vi "vipm_BuildVIPackage.vi"(8 "error in (no error)":errorcluster, 11 "CommandLine":string[](array[string])) -> (0 "error out":errorcluster, 2 "test details":string, 3 "output to action":string)   [LabVIEW 2014]
uses:
  <userlib>/_OpenG.lib/string/string.llb/Trim Whitespace (String)__ogtk.vi
  <vilib>/JKI/VIPM API/VIPM API_vipm_api.lvlib
  _lvcicd/_lvcicd_support_2014.lvlib
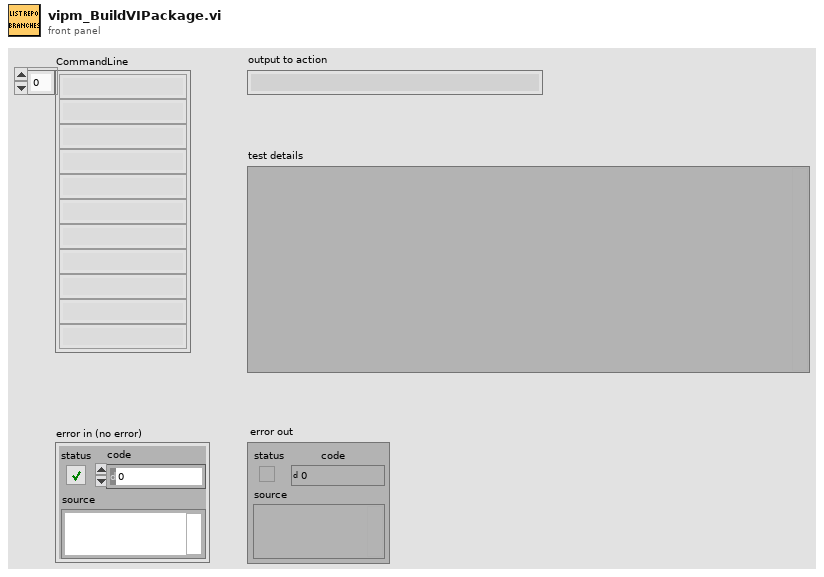
[diagram p1: front panel]
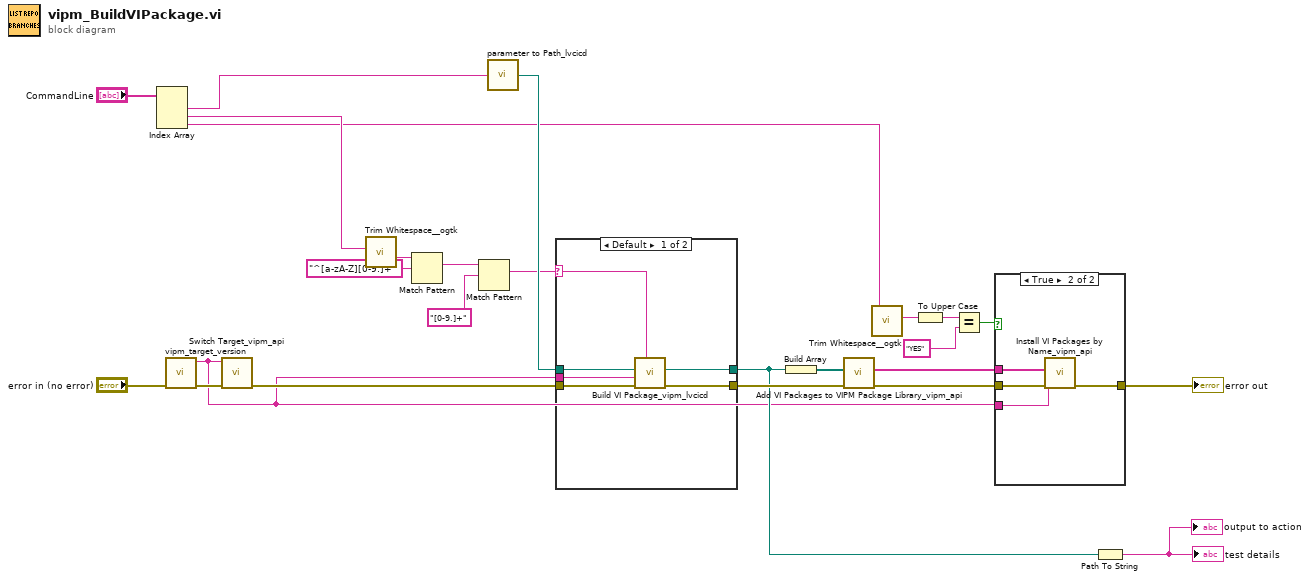
[diagram p0: block diagram]
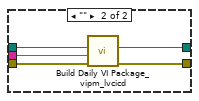
[diagram p2: hidden frame]
diagram:
  n1 = Index Array(array="CommandLine") -> (element #1=w22:string, element #2=w2:string, element #3=w1:string)  [unwired: 3 in]
  n2 = call "vipm_target_version.vi"() -> ("vipm Taget version"=w9:string)  [unwired: 11 in]
  n3 = call <vilib>:"Switch Target_vipm_api.vi"("error in (no error)"="error in (no error)", "LabVIEW Version"=w9) -> ("error out"=w10:errorcluster)  [unwired: 9 in]
  n4 = call-poly <userlib>:"Trim Whitespace__ogtk.vi"("String in"=w2) -> ("String out"=w7:string)  [unwired: 6 in]
  n5 = Match Pattern(string=w7, regular expression="^[a-zA-Z][0-9.]+") -> (match substring=w5:string)  [unwired: 1 in, 3 out]
  n6 = Match Pattern(string=w5, regular expression="[0-9.]+") -> (match substring=w3:string)  [unwired: 1 in, 3 out]
  n7 = call "parameter to Path_lvcicd.vi"("String"=w22) -> ("Path"=w24:path)
  n8 = case shown="Default" w3 {
    selector: w3 -> [w26 _]
    tunnel: w24 -> [w30 w35]
    tunnel: [w28 w34] -> w20
    tunnel: [w29 w33] -> w12
    tunnel: w10 -> [w27 w32]
    tunnel: w9 -> [w25 w31]
    frame Default {
      n9 = call "Build VI Package_vipm_lvcicd.vi"("Version string(x.x.x.x)"=w26, "error in (no error)"=w27, "LabVIEW Version"=w25, "vipb"=w30) -> ("error out"=w28:errorcluster, "Build Output"=w29:path)  [unwired: 4 in, 2 out]
    }
    frame "" {
      n10 = call "Build Daily VI Package_vipm_lvcicd.vi"("error in (no error)"=w32, "LabVIEW Version"=w31, "vipb"=w35) -> ("error out"=w34:errorcluster, "Build Output"=w33:path)  [unwired: 5 in, 2 out]
    }
  }
  n11 = Build Array(w12) -> (w21:path[])
  n12 = call <vilib>:"Add VI Packages to VIPM Package Library_vipm_api.vi"("error in (no error)"=w20, "Packages to add to VIPM Library (vipc,vip,ogp)"=w21) -> ("error out"=w19:errorcluster, "Package Names Added"=w18:string[])  [unwired: 8 in]
  n13 = call-poly <userlib>:"Trim Whitespace__ogtk.vi"("String in"=w1) -> ("String out"=w13:string)  [unwired: 6 in]
  n14 = To Upper Case(1:w13) -> (0:w14:string)
  n15 = Equal?(x=w14, y="YES") -> (x = y?=w16:bool)
  n16 = case shown="True" w16 {
    tunnel: w19 -> [w36 w40]
    tunnel: [w36 w39] -> w17
    tunnel: w9 -> [_ w38]
    tunnel: w18 -> [_ w37]
    frame False {
    }
    frame True {
      n17 = call <vilib>:"Install VI Packages by Name_vipm_api.vi"("error in (no error)"=w40, "LabVIEW Version"=w38, "Package Names to Install []"=w37) -> ("error out"=w39:errorcluster)  [unwired: 8 in]
    }
  }
  "error out" <- w17
  n18 = Path To String(path=w12) -> (string=→"test details" →"output to action":string)
